vi "get_grating_names.vi"(4 "error in (no error)":errorcluster, 7 "grating file":path) -> (0 "error out":errorcluster, 2 "grating names":string[](array[string]), 3 "grating file out":path)   [LabVIEW 2015]
uses:
  <vilib>/Utility/config.llb/NI_LVConfig.lvlib
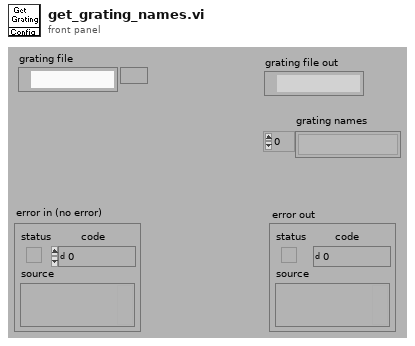
[diagram p1: front panel]
types:
  T1 = typedef "NI_LVConfig.lvlib/Config Data RefNum.ctl" = refnum<k1>
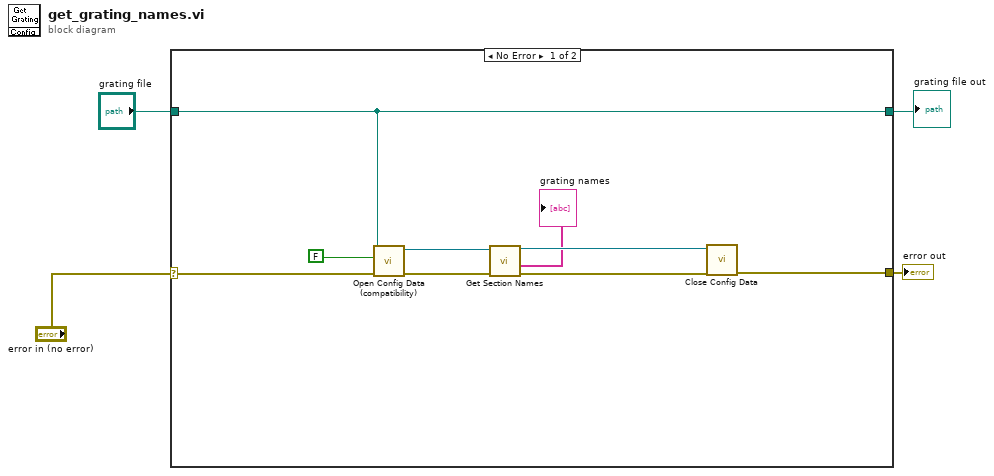
[diagram p0: block diagram]
diagram:
  n1 = case shown="No Error" "error in (no error)" {
    selector: "error in (no error)" -> [w5 w14]
    tunnel: [w11 w14] -> w4
    tunnel: "grating file" -> [w6 w15]
    tunnel: [w6 w15] -> w2
    frame No Error {
      n2 = call <vilib>:"Open Config Data (compatibility).vi"("error in (no error)"=w5, "create file if necessary (T)"=FALSE, "configuration file path"=w6) -> ("error out"=w12:errorcluster, "refnum"=w13:T1)  [unwired: 6 in, 1 out]
      n3 = call <vilib>:"Get Section Names.vi"("error in (no error)"=w12, "refnum"=w13) -> ("error out"=w9:errorcluster, "section names"=→"grating names":string[], "refnum out"=w8:T1)  [unwired: 7 in]
      n4 = call <vilib>:"Close Config Data.vi"("error in (no error)"=w9, "refnum"=w8) -> ("error out"=w11:errorcluster)  [unwired: 8 in, 1 out]
    }
    frame Error {
    }
  }
  "error out" <- w4
  "grating file out" <- w2
